vi "Position Numeric Input Field.vi"(8 "error in (no error)":errorcluster, 10 "Instruction String":refnum<vi>, 11 "Input field":refnum<vi>) -> (0 "error out":errorcluster)   [LabVIEW 2014]
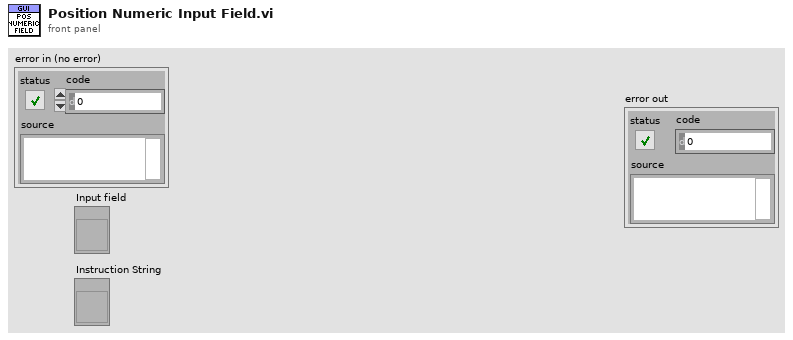
[diagram p1: front panel]
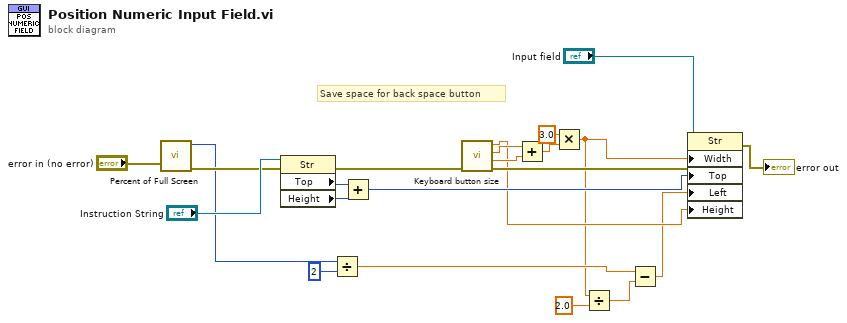
[diagram p0: block diagram]
diagram:
  # "Save space for back space button"
  n1 = call "Percent of Full Screen.vi"("error in (no error)"="error in (no error)") -> ("error out"=w18:errorcluster, "Right"=w7:i16)  [unwired: 8 in, 1 out]
  n2 = property class="Str"(reference="Instruction String", error in=w18) -> (error out=w17:errorcluster, "Top"=w20:i32, "Height"=w19:u32)  [unwired: 1 out]
  n3 = Divide(x=w7, y=i16 2) -> (x/y=w5:dbl)
  n4 = Add(x=w20, y=w19) -> (x+y=w12:u32)
  n5 = call "Keyboard button size.vi"("error in (no error)"=w17) -> ("error out"=w13:errorcluster, "Key Spacing"=w15:dbl, "Key Width"=w16:dbl, "Key Height"=w10:dbl)  [unwired: 7 in]
  n6 = Add(x=w16, y=w15) -> (x+y=w9:dbl)
  n7 = Multiply(x=3.0, y=w9) -> (x*y=w4:dbl)
  n8 = Divide(x=w4, y=2.0) -> (x/y=w2:dbl)
  n9 = Subtract(x=w5, y=w2) -> (x-y=w1:dbl)
  n10 = property class="Str"(reference="Input field", error in=w13, "Width"=w4, "Top"=w12, "Left"=w1, "Height"=w10) -> (error out=→"error out":errorcluster)  [unwired: 1 out]
